vi "Modbus_Comm_Tester.vi"(8 "error in (no error)":errorcluster, 9 "quantity":u16, 10 "starting address":u16) -> (0 "error out":errorcluster, 1 "Input _Registers":u16[](array[numeric]), 2 "Inputs":bool[](array[boolean]), 3 "Coils":bool[](array[boolean]))   [LabVIEW 2016]
uses:
  MB_Master_TCP/MB_Master_TCP.lvclass
  C:/Users/PRANAV/Desktop/Modbus_Scada_Main/Modbus_Scada/MB_Master/MB_Master.lvclass
  MB Master.lvlib
panel:
  in  "Timeout (10000) 2":i32=10000
  in  "Port (502) 2":u16=502
  in  "IP Address 2":string="localhost"
  # "Read Coils"
  # "Read Discrete Inputs"
  # "Read Input Registers"
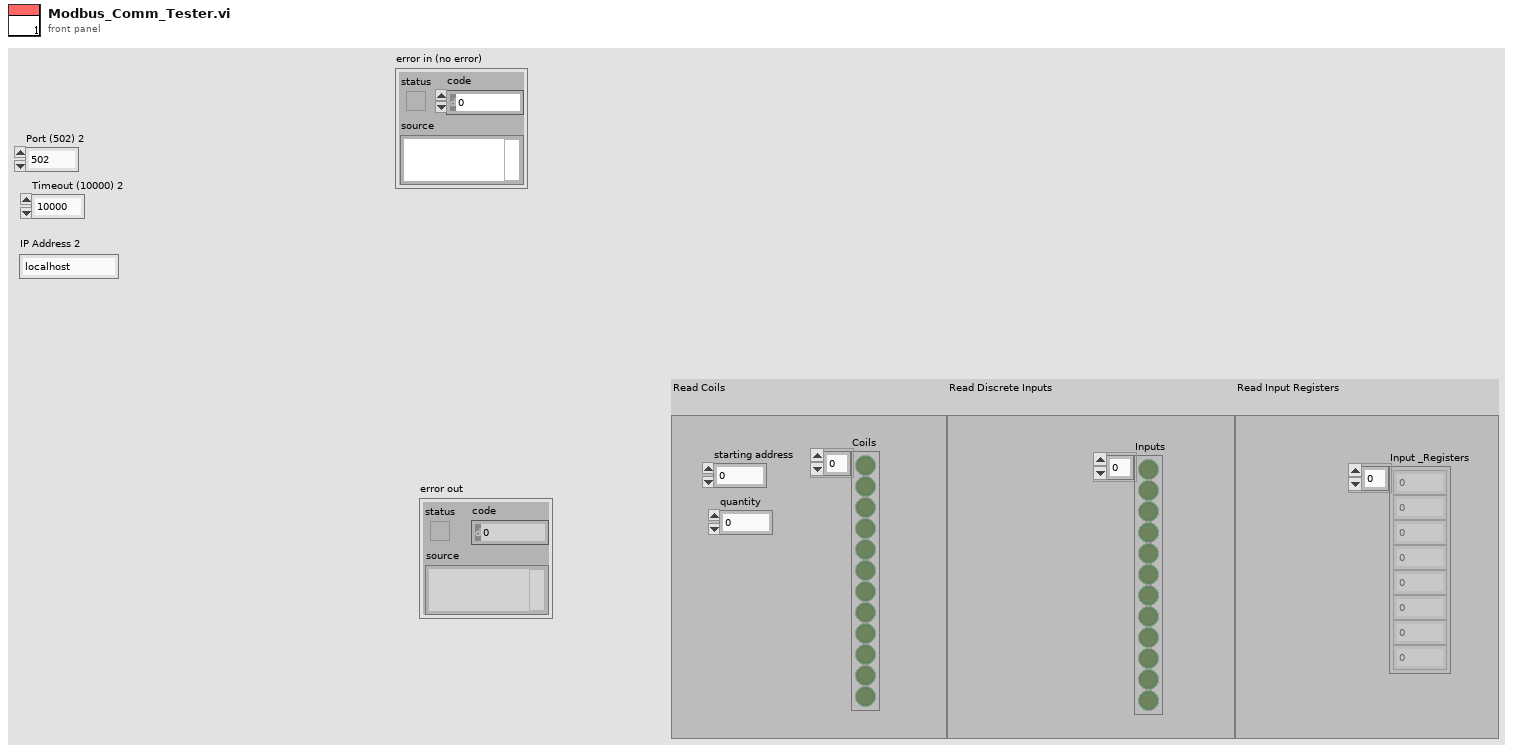
[diagram p1: front panel]
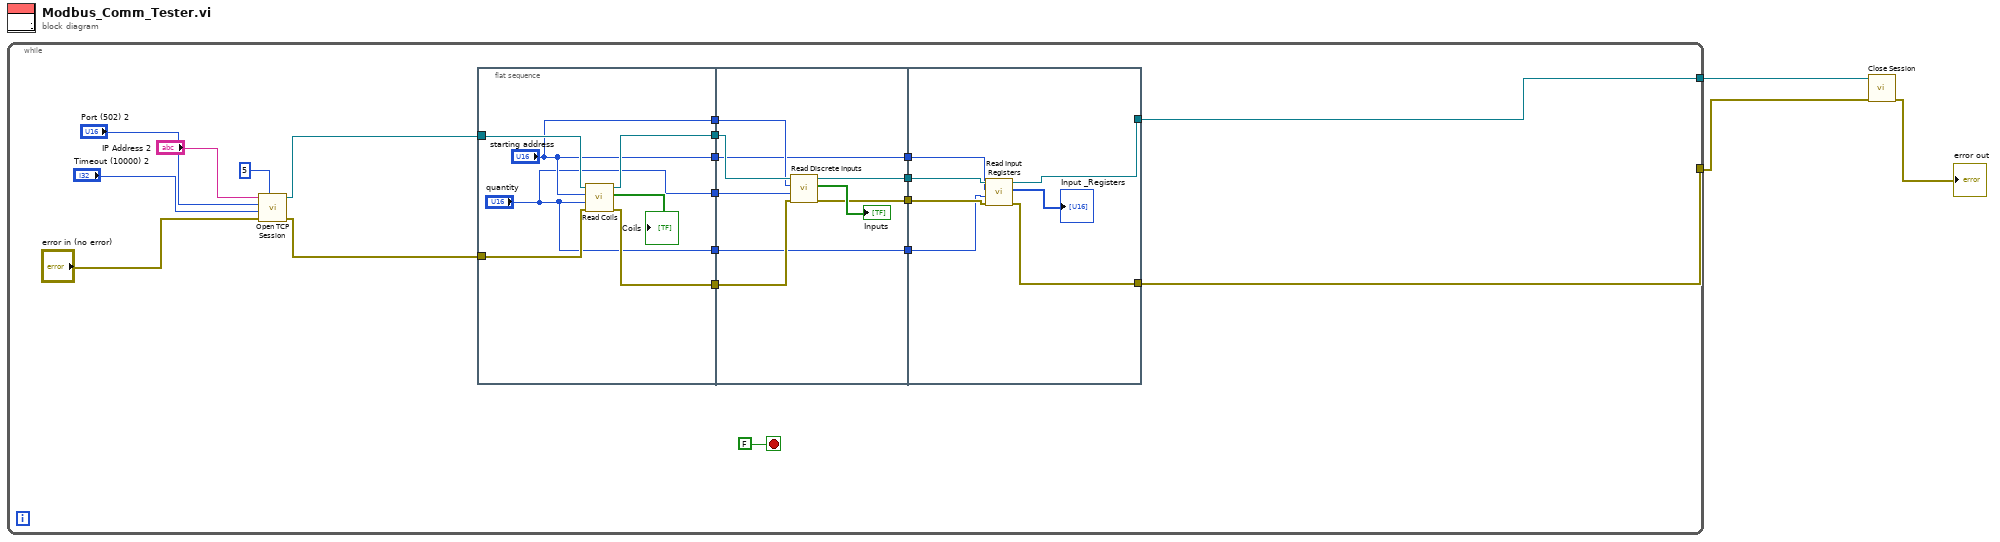
[diagram p0: block diagram]
diagram:
  n1 = while {
    tunnel: [w16] -> w2
    tunnel: [w15] -> w1
    stop <- FALSE stop-if-true
    n2 = call "Open TCP Session.vi"("Slave ID (255)"=u8 5, "error in (no error)"="error in (no error)", "Timeout (10000)"="Timeout (10000) 2", "Port (502)"="Port (502) 2", "IP Address"="IP Address 2") -> ("error out"=w10:errorcluster, "MB_TCP session"=w9:refnum<class "MB_Master_TCP.lvclass">)  [unwired: 5 in]
    n3 = flat-sequence {
      tunnel: w9 -> [w30]
      tunnel: w10 -> [w29]
      tunnel: [w27] -> w22
      tunnel: [w26] -> w21
      tunnel: ["starting address"] -> w20
      tunnel: ["quantity"] -> w19
      tunnel: ["starting address"] -> w6
      tunnel: ["quantity"] -> w4
      tunnel: w22 -> [w38]
      tunnel: w21 -> [w39]
      tunnel: w20 -> [w36]
      tunnel: w19 -> [w35]
      tunnel: [w34] -> w18
      tunnel: [w33] -> w17
      tunnel: [w32] -> w7
      tunnel: w6 -> [w32]
      tunnel: [w31] -> w5
      tunnel: w4 -> [w31]
      tunnel: w18 -> [w45]
      tunnel: w17 -> [w44]
      tunnel: [w43] -> w16
      tunnel: [w42] -> w15
      tunnel: w7 -> [w41]
      tunnel: w5 -> [w40]
      frame #0 {
        n4 = call "Read Coils.vi"("error in (no error)"=w29, "quantity"="quantity", "starting address"="starting address", "MB session in"=w30) -> ("error out"=w26:errorcluster, "Coils"=→"Coils":bool[], "MB session out"=w27:refnum<class "MB_Master_TCP.lvclass">)  [unwired: 5 in]
      }
      frame #1 {
        n5 = call "Read Discrete Inputs.vi"("error in (no error)"=w39, "quantity"=w35, "starting address"=w36, "MB session in"=w38) -> ("error out"=w33:errorcluster, "Inputs"=→"Inputs":bool[], "MB session out"=w34:refnum<class "MB_Master_TCP.lvclass">)  [unwired: 5 in]
      }
      frame #2 {
        n6 = call "Read Input Registers.vi"("error in (no error)"=w44, "quantity"=w40, "starting address"=w41, "MB session in"=w45) -> ("error out"=w42:errorcluster, "Registers"=→"Input _Registers":u16[], "MB session out"=w43:refnum<class "MB_Master_TCP.lvclass">)  [unwired: 5 in]
      }
    }
  }
  n7 = call-dynamic "Close Session.vi"("error in (no error)"=w1, "MB TCP session"=w2) -> ("error out"=→"error out":errorcluster)  [unwired: 9 in]
